vi "test適應性控制DAQmx API(實際控制).vi"() -> ()   [LabVIEW 2010]
uses:
  <vilib>/DAQmx/read.llb/DAQmx Read (Analog DBL 1Chan 1Samp).vi
  <vilib>/DAQmx/create/channels.llb/DAQmx Create Channel (AI-Voltage-Basic).vi
  <vilib>/DAQmx/configure/timing.llb/DAQmx Timing (Sample Clock).vi
  <vilib>/daqmx/miscellaneous.llb/DAQmx Fill In Error Info.vi
panel:
  in  "rate 2":dbl=1000.0 format="%0.2f"
  in  "samples per channel":i32=1000
  in  "timeout 2":dbl=10.0 format="%0.2f"
  in  "physical channels 2":tag
  in  "timeout":dbl=10.0 format="%0.2f"
  in  "physical channels":tag
  in  "number of samples":i32=100
  out "while 每次運行時間":u32
  in  "rate":dbl=1000.0
  out "收斂時間(s)":dbl
  out "收斂燈":bool
  in  "ERR誤差低於多少V亮燈":dbl=0.05
  out "ERR message":string=" INSTRUCTIONS:\r\rNormal Use:  When using subVIs that incorporate the error in/error out (or error I/O) structure, place this handler where you want to inform the user of an error, typically at the end of the I/O data path, as the last action of the program.  If the error in error? is ERROR, the handler creates a message describing the error and its source.  If the type of dialog = 1 (default), the message is displayed to the user, who can only acknowedge it.  If the type = 2, the user can acknowledge the message or abort execution; aborting a program with active I/O is not recommended.  If the type = 0, no message is displayed; this is used to process the error programmatically, and the error out cluster elements are wired to individual terminals for that reason.  \r\rOther Use:\n\r\nlocal testing.  To test the error code of a subVI or function that does not have the error I/O structure, you can wire its error code and a source string to the local error code and error source inputs.  If error in error? indicates no error and error code is not equal to 0, the local code and source are substituted for the error in values, and error? is set TRUE (ERROR)."
  out "理想系統與FIR輸出":cluster{dbl, dbl}(graph)
  out "system輸出":dbl
  out "input_x(t)":dbl(graph)
  out "ERR":dbl(graph)
  out "權重函數向量":dbl[](array[numeric])
  in  "order":i32=8
  out "LMS":dbl[](graph)
  out "FIR輸出":dbl
  in  "Stop Button":bool
  in  "u(收斂係數)":dbl=0.005
  # "A0:模擬輸入 pulse_output 2"
  # "A1:理想系統 pulse_output 1"
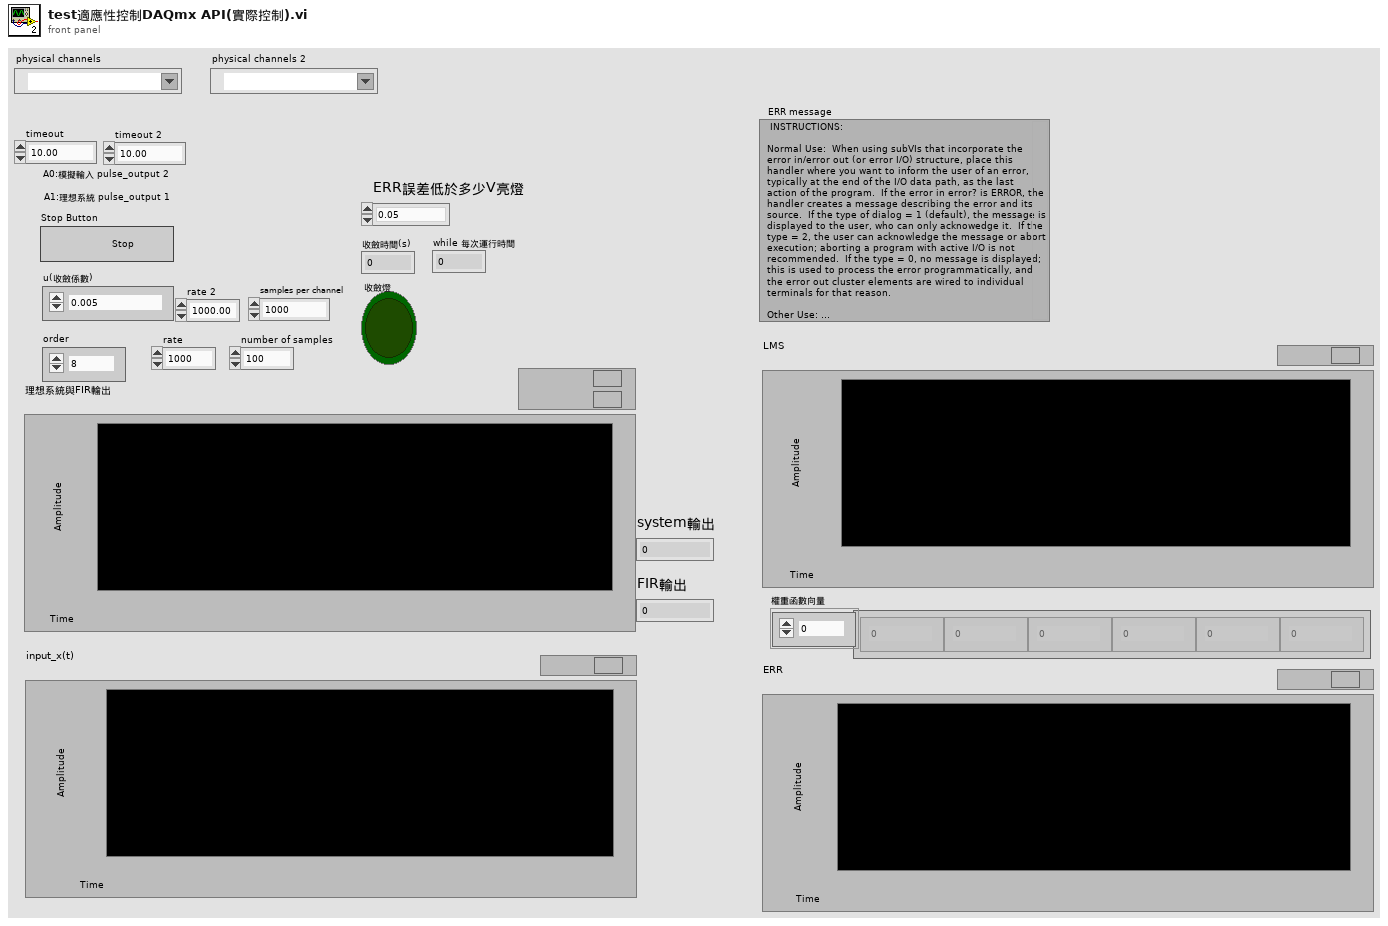
[diagram p1: front panel]
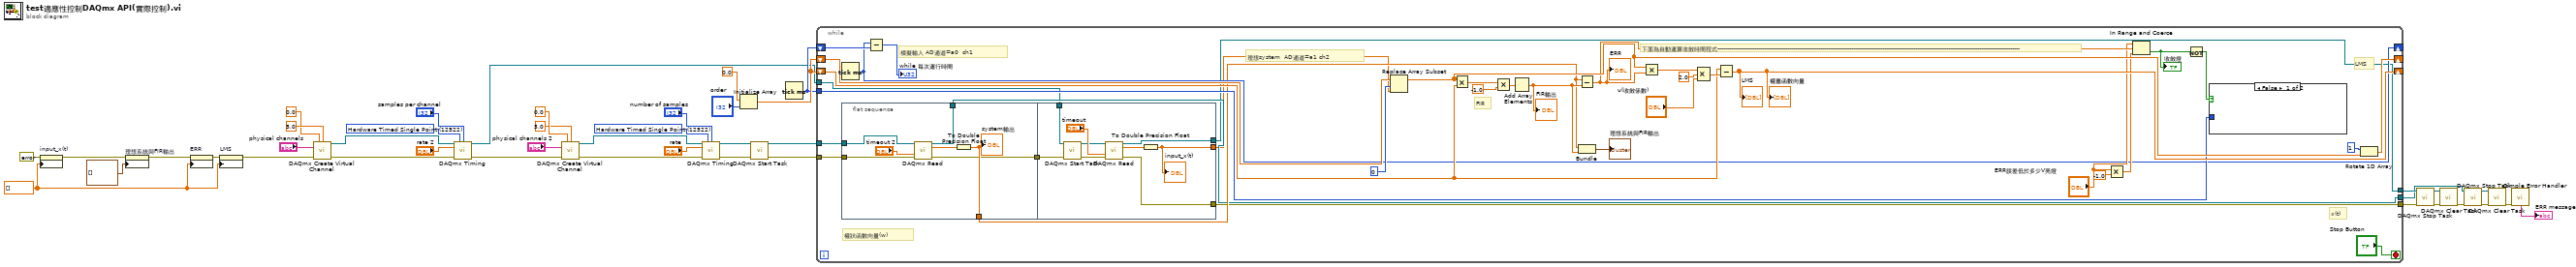
[diagram p0: block diagram]
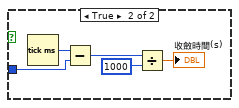
[diagram p2: hidden frame]
diagram:
  w18 = 12522 items=["Finite Samples"=10178, "Continuous Samples"=10123, "Hardware Timed Single Point"=12522] ("sample mode")
  w26 = 12522 items=["Finite Samples"=10178, "Continuous Samples"=10123, "Hardware Timed Single Point"=12522] ("sample mode")
  w39 = dbl[] [] ("History Data")
  n1 = property on="input_x(t)" class="WFChart (strict)"(error in=errorcluster {"status"=FALSE, "code"=0, "source"=""} ("error constant"), "History Data"=w39) -> (error out=w37:errorcluster)  [unwired: 1 in, 1 out]
  n2 = property on="理想系統與FIR輸出" class="WFChart (strict)"(error in=w37, "History Data"=cluster{dbl, dbl}[] []) -> (error out=w36:errorcluster)  [unwired: 1 in, 1 out]
  n3 = property on="ERR" class="WFChart (strict)"(error in=w36, "History Data"=w39) -> (error out=w38:errorcluster)  [unwired: 1 in, 1 out]
  n4 = property on="LMS" class="WFChart (strict)"(error in=w38, "History Data"=w39) -> (error out=w27:errorcluster)  [unwired: 1 in, 1 out]
  n5 = call-poly <vilib>:"DAQmx Create Virtual Channel.vi"("maximum value"=5.0, "minimum value"=0.0, "physical channels"="physical channels", "error in"=w27) -> ("task out"=w29:refnum<k21>, "error out"=w28:errorcluster)  [unwired: 10 in]
  n6 = call-poly <vilib>:"DAQmx Timing.vi"("task/channels in"=w29, "sample mode"=w26, "samples per channel"="samples per channel", "rate"="rate 2", "error in"=w28) -> ("task out"=w3:refnum<k21>, "error out"=w2:errorcluster)  [unwired: 9 in]
  n7 = call-poly <vilib>:"DAQmx Create Virtual Channel.vi"("maximum value"=5.0, "minimum value"=0.0, "physical channels"="physical channels 2", "error in"=w2) -> ("task out"=w16:refnum<k21>, "error out"=w23:errorcluster)  [unwired: 10 in]
  n8 = call-poly <vilib>:"DAQmx Timing.vi"("task/channels in"=w16, "sample mode"=w18, "samples per channel"="number of samples", "rate"="rate", "error in"=w23) -> ("task out"=w7:refnum<k21>, "error out"=w6:errorcluster)  [unwired: 9 in]
  n9 = Initialize Array "Initialize Array"(0.0 ("element"), "order") -> (w41:dbl[])
  n10 = call <vilib>:"DAQmx Start Task.vi"("task/channels in"=w7, "error in"=w6) -> ("task out"=w4:refnum<k21>, "error out"=w5:errorcluster)  [unwired: 12 in]
  n11 = Tick Count (ms)() -> (millisecond timer value=w33:u32)
  n12 = while {
    shift-right: [w70] -> _
    shift-left: w41 -> [w69]
    shift-right: [w66] -> _
    shift-left: w41 -> [w65]
    shift-right: [w54] -> _
    shift-left: w33 -> [w56]
    tunnel: w33 -> [w55]
    tunnel: [w47] -> w14
    tunnel: [w48] -> w13
    tunnel: w5 -> [w51]
    tunnel: w4 -> [w52]
    tunnel: w3 -> [w45]
    tunnel: [w49] -> w1
    stop <- "Stop Button" stop-if-true
    # "下面為自動運算收斂時間程式------------------------------------------------------------------------------------------------------------------------------------------------------------"
    # "LMS"
    # "FIR"
    # "模擬輸入 AD通道=a0  ch1"
    # "權狀函數向量(w)"
    # "x(t)"
    # "理想system  AD通道=a1 ch2"
    n13 = Tick Count (ms)() -> (millisecond timer value=w54:u32)
    n14 = flat-sequence {
      tunnel: w52 -> [w85]
      tunnel: w51 -> [w84]
      tunnel: [w82] -> w50
      tunnel: [w81] -> w49
      tunnel: [w80] -> w44
      tunnel: [w94] -> w48
      tunnel: [w93] -> w47
      tunnel: [w91] -> w46
      tunnel: w45 -> [w89]
      tunnel: w44 -> [w87]
      frame #0 {
        n15 = call-poly <vilib>:"DAQmx Read.vi"("task/channels in"=w85, "timeout"="timeout 2", "error in"=w84) -> ("task out"=w81:refnum<k21>, "data"=w83:dbl, "error out"=w80:errorcluster)  [unwired: 10 in]
        n16 = To Double Precision Float(number=w83) -> (double precision float=w82:dbl)
        "system輸出" <- w82
      }
      frame #1 {
        n17 = call <vilib>:"DAQmx Start Task.vi"("task/channels in"=w89, "error in"=w87) -> ("task out"=w90:refnum<k21>, "error out"=w88:errorcluster)  [unwired: 12 in]
        n18 = call-poly <vilib>:"DAQmx Read.vi"("task/channels in"=w90, "timeout"="timeout", "error in"=w88) -> ("task out"=w93:refnum<k21>, "data"=w92:dbl, "error out"=w94:errorcluster)  [unwired: 10 in]
        n19 = To Double Precision Float(number=w92) -> (double precision float=w91:dbl)
        "input_x(t)" <- w91
      }
    }
    n20 = Subtract(x=w54, y=w56) -> (x-y=→"while 每次運行時間":u32)
    n21 = Replace Array Subset "Replace Array Subset"(array=w69, new element=w46, index=0) -> (w67:dbl[])
    n22 = Multiply(x=w67, y=w65) -> (x*y=w79:dbl[])
    n23 = Multiply(x=w79, y=-1.0) -> (x*y=w72:dbl[])
    n24 = Add Array Elements(numeric array=w72) -> (sum=w64:dbl)
    "FIR輸出" <- w64
    n25 = Subtract(x=w50, y=w64) -> (x-y=w62:dbl)
    "ERR" <- w62
    n26 = Bundle(w50, w64) -> (→"理想系統與FIR輸出":cluster{dbl, dbl})  [unwired: 1 in]
    n27 = Multiply(x=w67, y=w62) -> (x*y=w77:dbl[])
    n28 = Compound Arithmetic op=MULTIPLY(w77, 2.0 ("value"), "u(收斂係數)") -> (w74:dbl[])
    n29 = Subtract(x=w65, y=w74) -> (x-y=w66:dbl[])
    "LMS" <- w66
    "權重函數向量" <- w66
    n30 = Multiply(x="ERR誤差低於多少V亮燈", y=-1.0) -> (x*y=w61:dbl)
    n31 = In Range and Coerce(upper limit="ERR誤差低於多少V亮燈", x=w62, lower limit=w61) -> (In Range?=w57:bool)  [unwired: 1 out]
    "收斂燈" <- w57
    n32 = Not(x=w57) -> (.not. x?=w58:bool)
    n33 = case shown="False" w58 {
      tunnel: w55 -> [_ w99]
      frame False {
      }
      frame True {
        n34 = Tick Count (ms)() -> (millisecond timer value=w100:u32)
        n35 = Subtract(x=w100, y=w99) -> (x-y=w98:u32)
        n36 = Divide(x=w98, y=u32 1000) -> (x/y=→"收斂時間(s)":dbl)
      }
    }
    n37 = Rotate 1D Array(1:w67, 2:1 ("n")) -> (0:w70:dbl[])
  }
  n38 = call <vilib>:"DAQmx Stop Task.vi"("task/channels in"=w14, "error in"=w13) -> ("task out"=w11:refnum<k21>, "error out"=w12:errorcluster)  [unwired: 12 in]
  n39 = call <vilib>:"DAQmx Clear Task.vi"("task in"=w11, "error in"=w12) -> ("error out"=w10:errorcluster)  [unwired: 13 in]
  n40 = call <vilib>:"DAQmx Stop Task.vi"("task/channels in"=w1, "error in"=w10) -> ("task out"=w15:refnum<k21>, "error out"=w9:errorcluster)  [unwired: 12 in]
  n41 = call <vilib>:"DAQmx Clear Task.vi"("task in"=w15, "error in"=w9) -> ("error out"=w8:errorcluster)  [unwired: 13 in]
  n42 = call <vilib>:"Simple Error Handler.vi"("error in (no error)"=w8) -> ("message"=→"ERR message":string)  [unwired: 4 in, 4 out]
